vi "Python Utility.vi"(6 "run minimized? (F)":bool, 7 "wait until completion? (T)":bool=TRUE, 8 "error in (no error)":errorcluster, 10 "Parameters String":string, 11 "Python Directory":path) -> (0 "error out":errorcluster, 1 "standard error":string, 2 "standard output":string)   [LabVIEW 2016, in "Webscraper.lvlib"]
doc: "This VI serves as a JFlash Command Prompt / CLI by accepting and passing command to JFlash.exe."
uses:
  Webscraper.lvlib
panel:
  out "return code":i32
  out "length":i32
  out "command line":string
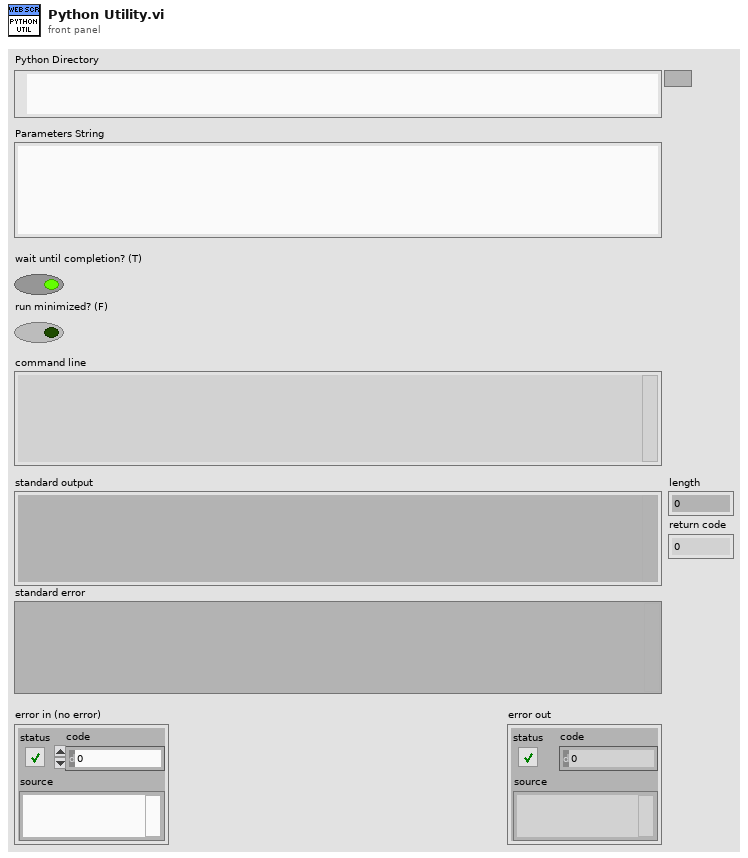
[diagram p1: front panel]
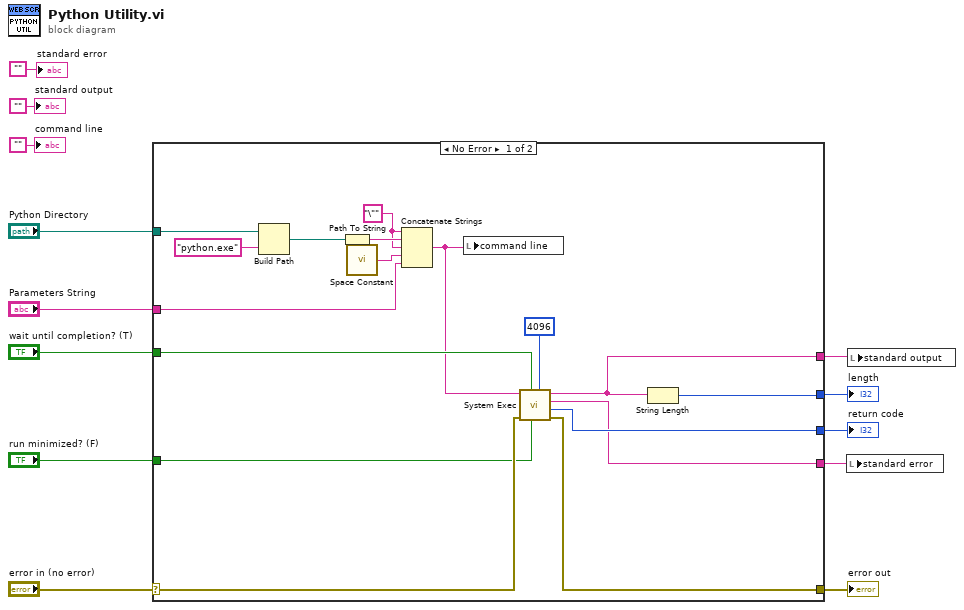
[diagram p0: block diagram]
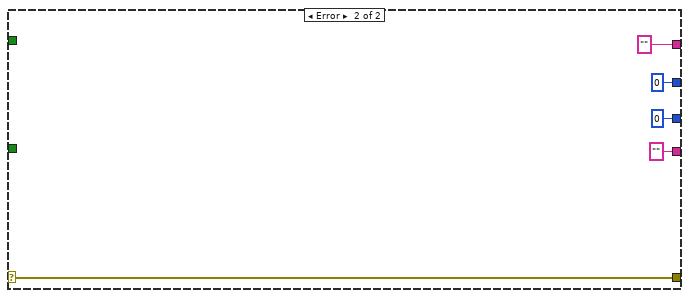
[diagram p2: hidden frame]
diagram:
  n1 = case shown="No Error" "error in (no error)" {
    selector: "error in (no error)" -> [w29 w35]
    tunnel: [w28 w35] -> w12
    tunnel: "Python Directory" -> [w20 _]
    tunnel: [w24 "" ("standard output")] -> w6
    tunnel: "wait until completion? (T)" -> [w26 _]
    tunnel: "run minimized? (F)" -> [w25 _]
    tunnel: "Parameters String" -> [w16 _]
    tunnel: [w23 0] -> w5
    tunnel: [w22 0 ("return code")] -> w4
    tunnel: [w14 "" ("standard error")] -> w2
    frame No Error {
      w17 = "\"" ("string")
      n2 = Build Path(base path=w20, name or relative path="python.exe" ("string")) -> (appended path=w18:path)
      n3 = Path To String(path=w18) -> (string=w30:string)
      n4 = call <vilib>:"Space Constant.vi"() -> ("String"=w15:string)
      n5 = Concatenate Strings(w17, w30, w17, w15, w16) -> (w21:string)
      n6 = local write "command line"(w21) -> ()
      n7 = call <vilib>:"System Exec.vi"("expected output size  (4096)"=u32 4096, "run minimized? (F)"=w25, "wait until completion? (T)"=w26, "error in (no error)"=w29, "command line"=w21) -> ("error out"=w28:errorcluster, "return code"=w22:i32, "standard error"=w14:string, "standard output"=w24:string)  [unwired: 3 in]
      n8 = String Length(string=w24) -> (length=w23:i32)
    }
    frame Error {
    }
  }
  "error out" <- w12
  "length" <- w5
  "return code" <- w4
  n9 = local write "standard error"(w2) -> ()
  n10 = local write "standard output"(w6) -> ()
  "standard output" <- ""
  "command line" <- ""
  "standard error" <- ""
